vi "测试.vi"() -> ()   [LabVIEW 2018]
panel:
  in  "路径 3":path=path "E:/登陆系统重写/dist/predict"
  in  "路径 2":path=path "E:/登陆系统重写/保存文件路径.txt"
  in  "路径":path=path "E:/登陆系统重写/待检测文件路径.txt"
  in  "取消按钮":bool
  in  "确定按钮":bool
  in  "保存文件路径":path
  in  "待检测文件":path
  # "ME-NBI病变图像路径选择"
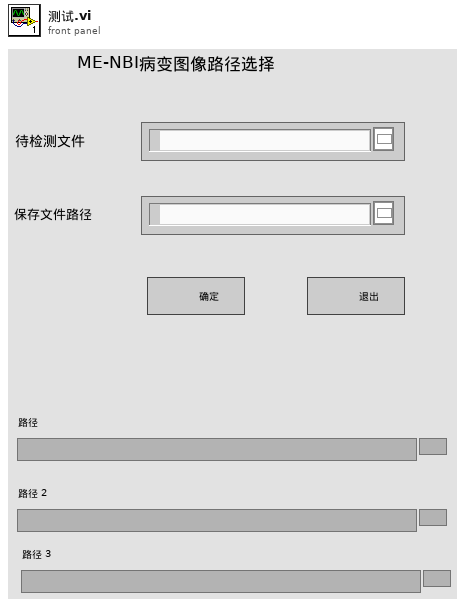
[diagram p1: front panel]
types:
  T1 = enum16{"open", "replace", "create", "open or create", "replace or create", "replace or create with confirmation"}
  T2 = enum32{"Invalid", "Standard", "Closed", "Hidden", "Minimized", "Maximized"}
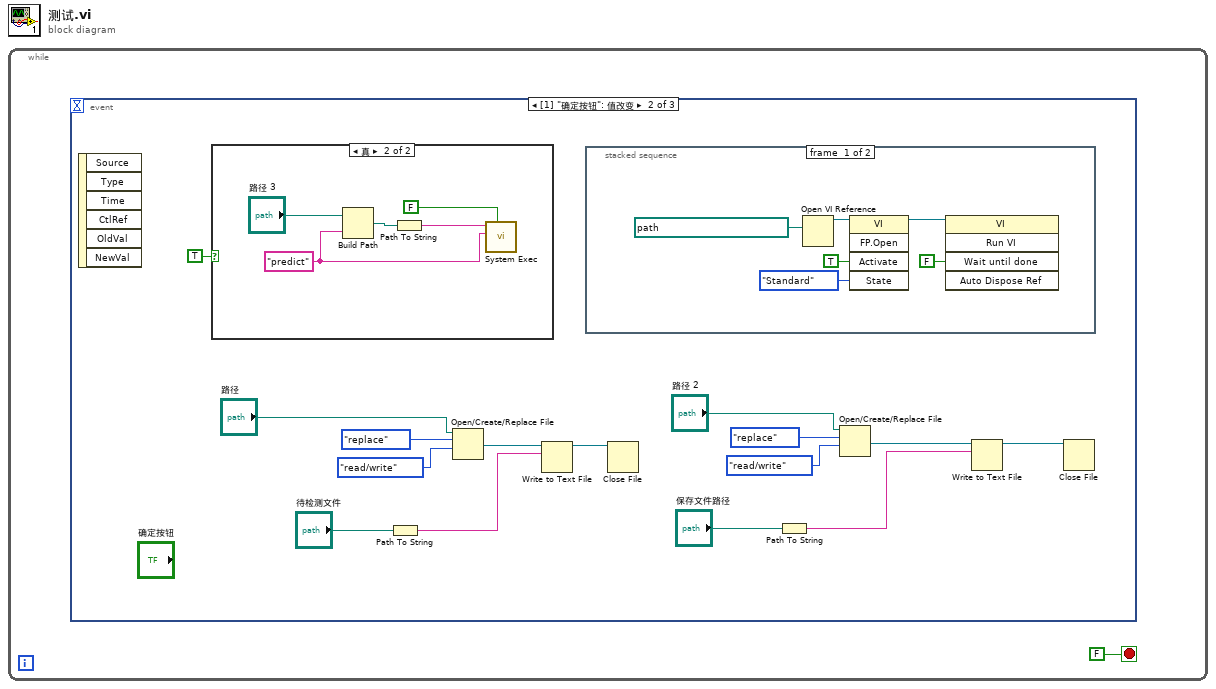
[diagram p0: block diagram]
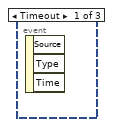
[diagram p2: hidden frame]
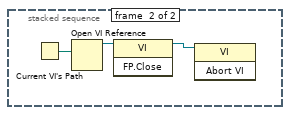
[diagram p4: hidden frame]
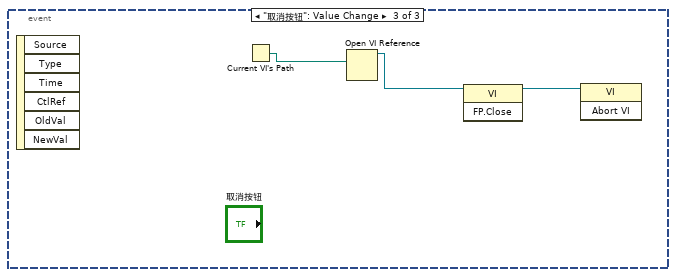
[diagram p5: hidden frame]
diagram:
  n1 = while {
    stop <- FALSE stop-if-true
    n2 = event shown="[1] \"确定按钮\": 值改变" {
      selector: _ -> [_ _ _]
      dyn-events: _ -> [_ _ _]
      timeout: _ -> [_ _ _]
      event Timeout {
        n3 = event-data() -> ()  [unwired: 1 in, 3 out]
      }
      event "确定按钮": Value Change {
        n4 = event-data() -> ()  [unwired: 1 in, 6 out]
        n5 = case shown="真" TRUE {
          frame False {
          }
          frame True {
            w17 = "predict" ("名称或相对路径")
            n6 = Build Path(base path="路径 3", name or relative path=w17) -> (appended path=w19:path)
            n7 = Path To String(path=w19) -> (string=w20:string)
            n8 = call <vilib>:"System Exec.vi"("wait until completion? (T)"=FALSE, "standard input"=w17, "command line"=w20) -> ()  [unwired: 5 in, 4 out]
          }
        }
        n9 = Path To String(path="待检测文件") -> (string=w11:string)
        n10 = Open/Create/Replace File(file path (use dialog)="路径", operation (0:open)=T1."replace" ("操作(0:open)"), access (0:read/write)=enum16{"read/write", "read-only", "write-only"}."read/write" ("权限(0:read/write)")) -> (refnum out=w13:refnum<file>)  [unwired: 3 in, 2 out]
        n11 = Write to Text File(file (use dialog)=w13, text=w11) -> (refnum out=w12:refnum<file>)  [unwired: 2 in, 2 out]
        n12 = stacked-sequence {
          frame #0 {
            n13 = Open VI Reference(vi path=path "E:/登陆系统重写/进度条.vi" ("VI路径")) -> (vi reference=w27:refnum<vi>)  [unwired: 5 in, 1 out]
            n14 = invoke class="VI" method="FP.Open"(reference=w27, "Activate"=TRUE ("激活？"), "State"=T2."Standard" ("状态")) -> (reference out=w26:refnum<vi>)  [unwired: 2 in, 4 out]
            n15 = invoke class="VI" method="Run VI"(reference=w26, "Wait until done"=FALSE ("结束前等待")) -> ()  [unwired: 3 in, 5 out]
          }
          frame #1 {
            n16 = Current VI's Path() -> (path=w30:path)
            n17 = Open VI Reference(vi path=w30) -> (vi reference=w29:refnum<vi>)  [unwired: 5 in, 1 out]
            n18 = invoke class="VI" method="FP.Close"(reference=w29) -> (reference out=w28:refnum<vi>)  [unwired: 2 in, 2 out]
            n19 = invoke class="VI" method="Abort VI"(reference=w28) -> ()  [unwired: 2 in, 3 out]
          }
        }
        n20 = Close File(refnum=w12) -> ()  [unwired: 1 in, 2 out]
        n21 = Path To String(path="保存文件路径") -> (string=w7:string)
        n22 = Open/Create/Replace File(file path (use dialog)="路径 2", operation (0:open)=T1."replace" ("操作(0:open)"), access (0:read/write)=enum16{"read/write", "read-only", "write-only"}."read/write" ("权限(0:read/write)")) -> (refnum out=w9:refnum<file>)  [unwired: 3 in, 2 out]
        n23 = Write to Text File(file (use dialog)=w9, text=w7) -> (refnum out=w8:refnum<file>)  [unwired: 2 in, 2 out]
        n24 = Close File(refnum=w8) -> ()  [unwired: 1 in, 2 out]
      }
      event "取消按钮": Value Change {
        n25 = event-data() -> ()  [unwired: 1 in, 6 out]
        n26 = Current VI's Path() -> (path=w33:path)
        n27 = Open VI Reference(vi path=w33) -> (vi reference=w32:refnum<vi>)  [unwired: 5 in, 1 out]
        n28 = invoke class="VI" method="FP.Close"(reference=w32) -> (reference out=w31:refnum<vi>)  [unwired: 2 in, 2 out]
        n29 = invoke class="VI" method="Abort VI"(reference=w31) -> ()  [unwired: 2 in, 3 out]
      }
    }
  }
